vi "Title.vi"(5 "Table Configuration":T1={"Table Settings"={"Number of Columns"=1, "Width (%)"=100.0, "Relative Column Widths (%)"=[100.0], "Horizontal Align"=0, "Header Rows"=0}, "Cell Defaults"={"Background Color"=16777215, "Horizontal Align"=3, "Vertical Align"=1, "Minimum Height"=0.0, "Fixed Height"=0.0, "Padding"={"Left"=2.0, "Top"=2.0, "Right"=2.0, "Bottom"=3.0}}, "Borders"={"Left"={"Enabled"=FALSE, "Width"=1.0, "Color"=16777215}, "Top"={"Enabled"=FALSE, "Width"=1.0, "Color"=16777215}, "Right"={"Enabled"=FALSE, "Width"=1.0, "Color"=16777215}, "Bottom"={"Enabled"=FALSE, "Width"=1.0, "Color"=16777215}, "Middle Horizontal"={"Enabled"=FALSE, "Width"=0.5, "Color"=16777215}, "Middle Vertical"={"Enabled"=FALSE, "Width"=0.5, "Color"=16777215}}} {"Cell Defaults"."Vertical Align" items=["Bottom", "Middle", "Top"]; "Cell Defaults"."Horizontal Align" items=["Center", "Justified", "JustifiedAll", "Left", "Right"]; "Table Settings"."Horizontal Align" items=["Center"=0, "Left"=3, "Right"=4]}, 6 "Add Line Feeds (F:No)":bool=TRUE, 7 "Cell Configuration":T5={"Cell Defaults"={"Background Color"=16777215, "Horizontal Align"=3, "Vertical Align"=1, "Minimum Height"=0.0, "Fixed Height"=0.0, "Padding"={"Left"=2.0, "Top"=2.0, "Right"=2.0, "Bottom"=3.0}}, "Borders"={"Left"={"Enabled"=FALSE, "Width"=1.0, "Color"=0}, "Top"={"Enabled"=FALSE, "Width"=1.0, "Color"=0}, "Right"={"Enabled"=FALSE, "Width"=1.0, "Color"=0}, "Bottom"={"Enabled"=FALSE, "Width"=1.0, "Color"=0}}, "Column Span"=0} {"Cell Defaults"."Vertical Align" items=["Bottom", "Middle", "Top"]; "Cell Defaults"."Horizontal Align" items=["Center", "Justified", "JustifiedAll", "Left", "Right"]}, 8 "error in (no error)":errorcluster, 9 "Font":T6={"Font"="Arial", "Size"=26, "Colour"=0, "Bold"=TRUE, "Italic"=FALSE, "Underline"=TRUE, "Strikethrough"=FALSE, "Font Encoding"=enum."Cp1252, WinANSI"}, 10 "Text":string="Test Result Sheet", 11 "Context in":refnum<class "Context.lvclass">) -> (0 "error out":errorcluster, 3 "Context out":refnum<class "Context.lvclass">)   [LabVIEW 2020, in "PDF Interface.lvlib" / "PDF Interface Helper.lvlib"]
doc: "Adds the title text into the PDF test report."
uses:
  PDF Interface Helper.lvlib
  <vilib>/Simplicity AI/SAI_PDF_API/Classes/Context/Controls/SAI_PDF_Font.ctl
  <vilib>/Simplicity AI/SAI_PDF_API/Classes/Context/Controls/SAI_PDF_Font Encoding.ctl
  <vilib>/Simplicity AI/SAI_PDF_API/Classes/Context/Context.lvclass
  <vilib>/Simplicity AI/SAI_PDF_API/Classes/Table Builder/Controls/SAI_PDF_Cell Configuration.ctl
  <vilib>/Simplicity AI/SAI_PDF_API/Classes/Table Builder/Controls/SAI_PDF_Default Cell Format.ctl
  <vilib>/Simplicity AI/SAI_PDF_API/Classes/Table Builder/Controls/SAI_PDF_BorderLine.ctl
  <vilib>/Simplicity AI/SAI_PDF_API/Classes/Table Builder/Controls/SAI_PDF_Table Configuration.ctl
  <vilib>/Simplicity AI/SAI_PDF_API/Classes/Table Builder/Controls/SAI_PDF_Table Horizontal Align.ctl
  <vilib>/Simplicity AI/SAI_PDF_API/Classes/Context/Controls/SAI_PDF_Text Align.ctl
  <vilib>/Simplicity AI/SAI_PDF_API/Classes/Table Builder/Table Builder.lvclass
  <vilib>/Simplicity AI/SAI_PDF_API/Classes/Context/Methods/Public/Low Level/Add/SAI_PDF_Add Paragraph.vi
panel:
  # "(Cp1252)"
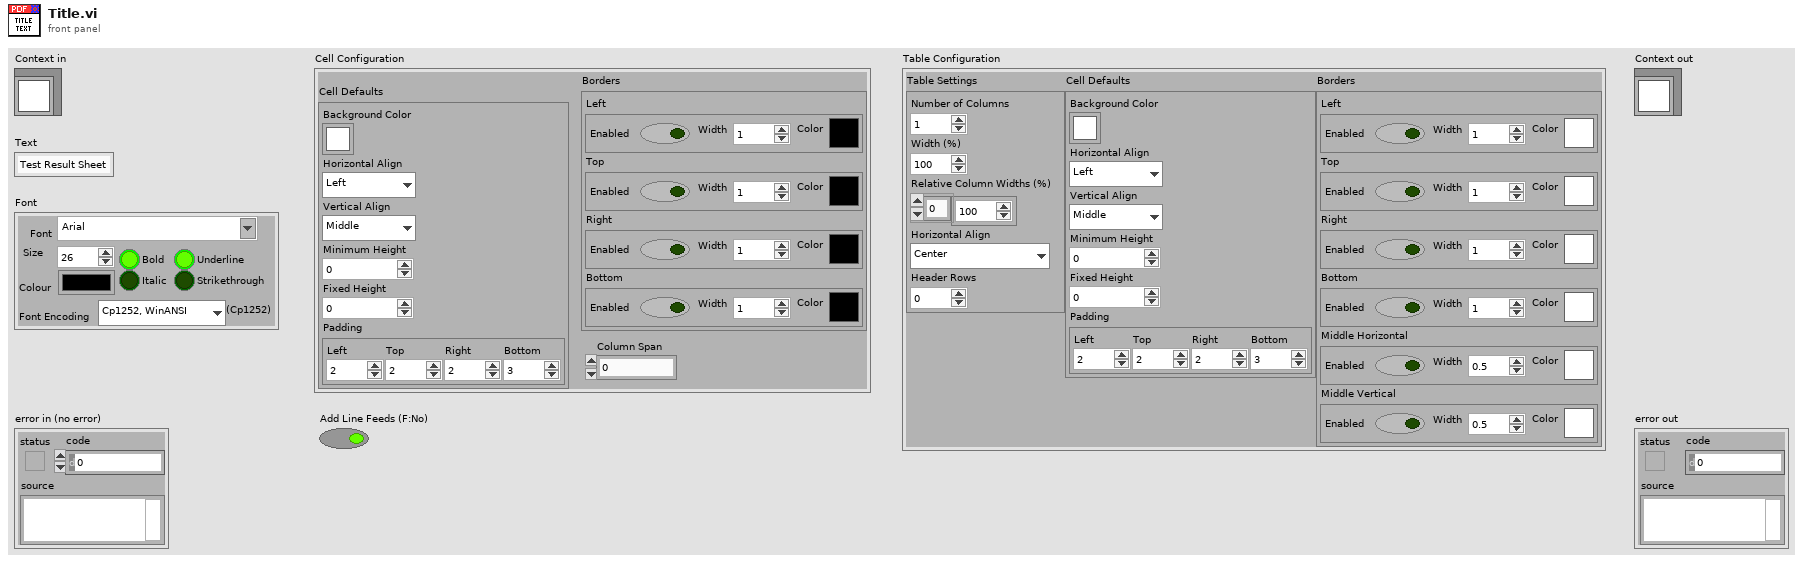
[diagram p1: front panel]
types:
  T1 = typedef "SAI_PDF_Toolkit.lvlib/Table Builder.lvclass/SAI_PDF_Table Configuration.ctl" = cluster{"Table Settings":cluster{"Number of Columns":i32, "Width (%)":sgl, "Relative Column Widths (%)":sgl[], "Horizontal Align":T2, "Header Rows":i32}, "Cell Defaults":T3, "Borders":cluster{"Left":T4, "Top":T4, "Right":T4, "Bottom":T4, "Middle Horizontal":T4, "Middle Vertical":T4}}
  T2 = typedef "SAI_PDF_Toolkit.lvlib/Table Builder.lvclass/SAI_PDF_Table Horizontal Align.ctl" = i32
  T3 = typedef "SAI_PDF_Toolkit.lvlib/Table Builder.lvclass/SAI_PDF_Default Cell Format.ctl" = cluster{"Background Color":u32, "Horizontal Align":i32, "Vertical Align":i32, "Minimum Height":sgl, "Fixed Height":sgl, "Padding":cluster{"Left":sgl, "Top":sgl, "Right":sgl, "Bottom":sgl}}
  T4 = typedef "SAI_PDF_Toolkit.lvlib/Table Builder.lvclass/SAI_PDF_BorderLine.ctl" = cluster{"Enabled":bool, "Width":sgl, "Color":u32}
  T5 = typedef "SAI_PDF_Toolkit.lvlib/Table Builder.lvclass/SAI_PDF_Cell Configuration.ctl" = cluster{"Cell Defaults":T3, "Borders":cluster{"Left":T4, "Top":T4, "Right":T4, "Bottom":T4}, "Column Span":i32}
  T6 = typedef "SAI_PDF_Toolkit.lvlib/Context.lvclass/SAI_PDF_Font.ctl" = cluster{"Font":string, "Size":i32, "Colour":u32, "Bold":bool, "Italic":bool, "Underline":bool, "Strikethrough":bool, "Font Encoding":T7}
  T7 = typedef "SAI_PDF_Toolkit.lvlib/Context.lvclass/SAI_PDF_Font Encoding.ctl" = enum16{"Cp1252, WinANSI", "IdentityH", "IdentityV", "Cp1250", "Cp1257", "MacRoman"}
  T8 = typedef "SAI_PDF_Toolkit.lvlib/Context.lvclass/SAI_PDF_Text Align.ctl" = i32
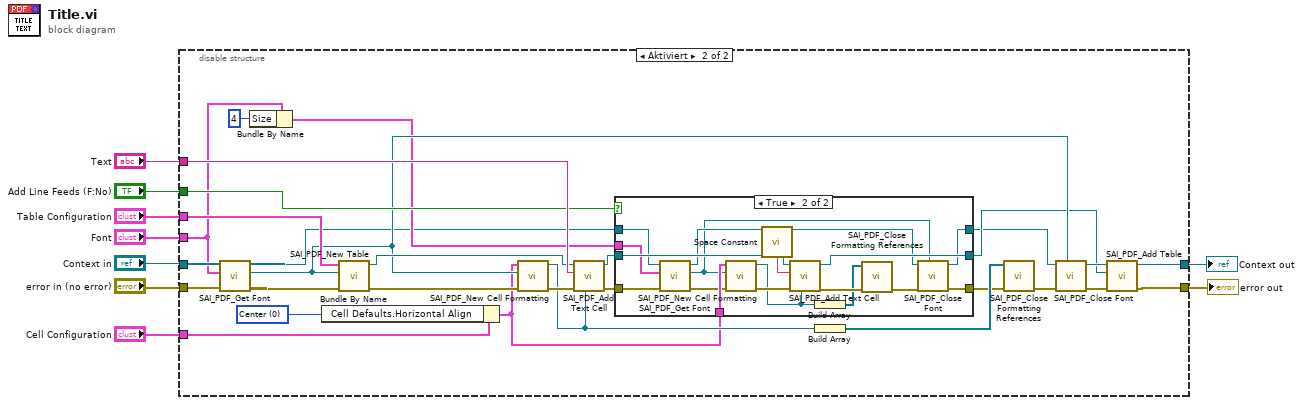
[diagram p0: block diagram]
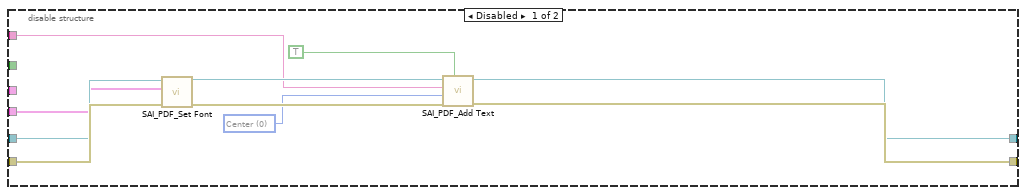
[diagram p2: hidden frame]
diagram:
  n1 = disable-structure shown="Aktiviert" {
    disable-tunnel: [w19 w44] -> w9
    disable-tunnel: [w18 w45] -> w8
    disable-tunnel: "error in (no error)" -> [w15 w46]
    disable-tunnel: "Context in" -> [w14 w47]
    disable-tunnel: "Font" -> [w13 w25]
    disable-tunnel: "Text" -> [w11 w48]
    disable-tunnel: "Cell Configuration" -> [_ w43]
    disable-tunnel: "Table Configuration" -> [_ w42]
    disable-tunnel: "Add Line Feeds (F:No)" -> [_ w41]
    frame Disabled {
      w12 = T8 0 items=["Center", "Justified", "Justified All", "Left", "Right"] ("Align (Left)")
      n2 = call <vilib>:"SAI_PDF_Set Font.vi"("error in"=w15, "Font"=w13, "Context In"=w14) -> ("error out"=w16:errorcluster, "Context Out"=w17:refnum<class "Context.lvclass">)  [unwired: 7 out]
      n3 = call-poly <vilib>:"SAI_PDF_Add Text.vi"("Add Line Feeds (F:No)"=TRUE, "error in"=w16, "Align (Left)"=w12, "Text"=w11, "Context In"=w17) -> ("error out"=w19:errorcluster, "Context Out"=w18:refnum<class "Context.lvclass">)  [unwired: 5 out]
    }
    frame Enabled {
      w26 = 0 items=["Center", "Justified", "JustifiedAll", "Left", "Right"] ("Horizontal Align")
      n4 = call <vilib>:"SAI_PDF_Get Font.vi"("error in"=w46, "Font"=w25, "Context In"=w47) -> ("error out"=w39:errorcluster, "Font"=w34:refnum<class "Font.lvclass">, "Context Out"=w21:refnum<class "Context.lvclass">)  [unwired: 6 out]
      n5 = Bundle By Name(cluster=w25, "Size"=4) -> (w23:T6)
      n6 = Bundle By Name(cluster=w43, "Cell Defaults.Horizontal Align"=w26) -> (w22:T5)
      n7 = call <vilib>:"SAI_PDF_New Table.vi"("error in"=w39, "Font In"=w34, "Table Configuration"=w42) -> ("error out"=w40:errorcluster, "Table Builder"=w37:refnum<class "Table Builder.lvclass">)  [unwired: 7 out]
      n8 = call <vilib>:"SAI_PDF_New Cell Formatting.vi"("error in"=w40, "Font In"=w34, "Cell Configuration"=w22) -> ("error out"=w38:errorcluster, "Cell Formatting"=w27:refnum<class "Formatting.lvclass">)  [unwired: 7 out]
      n9 = call <vilib>:"SAI_PDF_Add Text Cell.vi"("Formatting In"=w27, "error in"=w38, "Text"=w48, "Table Builder In"=w37) -> ("error out"=w31:errorcluster, "Table Builder Out"=w29:refnum<class "Table Builder.lvclass">)  [unwired: 6 in]
      n10 = case shown="True" w41 {
        tunnel: w31 -> [w50 w64]
        tunnel: [w50 w58] -> w30
        tunnel: w29 -> [w51 w66]
        tunnel: [w51 w67] -> w28
        tunnel: w21 -> [w49 w65]
        tunnel: w23 -> [_ w63]
        tunnel: w22 -> [_ w62]
        tunnel: [w49 w56] -> w20
        frame False {
        }
        frame True {
          n11 = call <vilib>:"SAI_PDF_Get Font.vi"("error in"=w64, "Font"=w63, "Context In"=w65) -> ("error out"=w61:errorcluster, "Font"=w57:refnum<class "Font.lvclass">, "Context Out"=w59:refnum<class "Context.lvclass">)  [unwired: 6 out]
          n12 = call <vilib>:"SAI_PDF_New Cell Formatting.vi"("error in"=w61, "Font In"=w57, "Cell Configuration"=w62) -> ("error out"=w60:errorcluster, "Cell Formatting"=w53:refnum<class "Formatting.lvclass">)  [unwired: 7 out]
          n13 = call <vilib>:"Space Constant.vi"() -> ("String"=w68:string)
          n14 = call <vilib>:"SAI_PDF_Add Text Cell.vi"("Formatting In"=w53, "error in"=w60, "Text"=w68, "Table Builder In"=w66) -> ("error out"=w55:errorcluster, "Table Builder Out"=w67:refnum<class "Table Builder.lvclass">)  [unwired: 6 in]
          n15 = Build Array(w53) -> (w52:refnum<class "Formatting.lvclass">[])
          n16 = call <vilib>:"SAI_PDF_Close Formatting References.vi"("error in"=w55, "Formatting Refs"=w52) -> ("error out"=w54:errorcluster)  [unwired: 9 out]
          n17 = call <vilib>:"SAI_PDF_Close Font.vi"("Font"=w57, "error in"=w54, "Context In"=w59) -> ("error out"=w58:errorcluster, "Context Out"=w56:refnum<class "Context.lvclass">)  [unwired: 7 out]
        }
      }
      n18 = Build Array(w27) -> (w36:refnum<class "Formatting.lvclass">[])
      n19 = call <vilib>:"SAI_PDF_Close Formatting References.vi"("error in"=w30, "Formatting Refs"=w36) -> ("error out"=w35:errorcluster)  [unwired: 9 out]
      n20 = call <vilib>:"SAI_PDF_Close Font.vi"("Font"=w34, "error in"=w35, "Context In"=w20) -> ("error out"=w32:errorcluster, "Context Out"=w33:refnum<class "Context.lvclass">)  [unwired: 7 out]
      n21 = call <vilib>:"SAI_PDF_Add Table.vi"("error in"=w32, "Table Builder In"=w28, "Context In"=w33) -> ("error out"=w44:errorcluster, "Context Out"=w45:refnum<class "Context.lvclass">)  [unwired: 7 out]
    }
  }
  "error out" <- w9
  "Context out" <- w8
